vi "MTM2_getSample_actuatorLimitSwitches.vi"(8 "error in (no error)":errorcluster, 11 "actuatorLimitSwitches_Ctl":T1) -> (0 "error out":errorcluster, 2 "function return":i32, 3 "actuatorLimitSwitches_Ctl out":T1)   [LabVIEW 2018, in "SALLV_MTM2.lvlib"]
doc: "int MTM2_shm_getSample_actuatorLimitSwitchesLV(MTM2_actuatorLimitSwitchesLV *actuatorLimitSwitches_Ctl );"
uses:
  SALLV_MTM2.lvlib
  DataTypes/actuatorLimitSwitches.ctl
  SALLV_MTM2.so
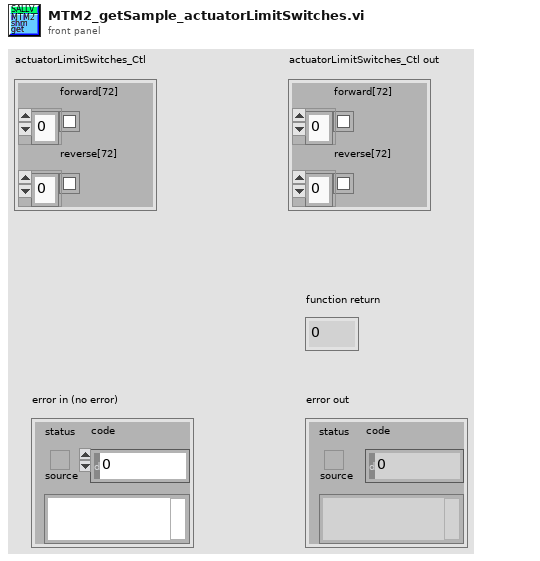
[diagram p1: front panel]
types:
  T1 = typedef "SALLV_MTM2.lvlib/actuatorLimitSwitches.ctl" = cluster{"forward[72]":bool[], "reverse[72]":bool[]}
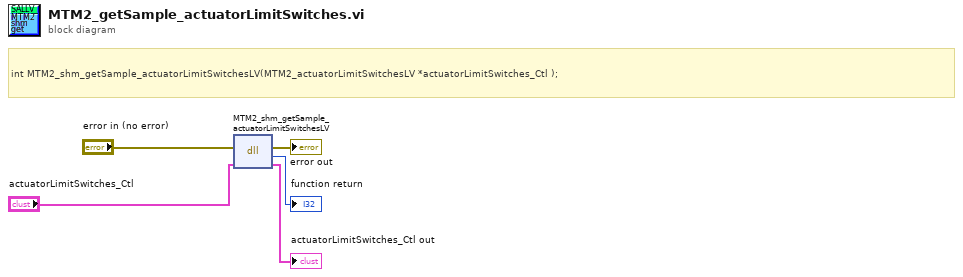
[diagram p0: block diagram]
diagram:
  # "int MTM2_shm_getSample_actuatorLimitSwitchesLV(MTM2_actuatorLimitSwitchesLV *actuatorLimitSwitches_Ctl );"
  n1 = dll-call lib="home/ttsai/Document/salApiMTM2/SALLV_MTM2/SALLV_MTM2.*" fn="MTM2_shm_getSample_actuatorLimitSwitchesLV"(error in="error in (no error)", "actuatorLimitSwitches_Ctl"="actuatorLimitSwitches_Ctl") -> (error out=→"error out":errorcluster, →"function return":i32, "actuatorLimitSwitches_Ctl"=→"actuatorLimitSwitches_Ctl out":T1)  [unwired: 2 in, 1 out]
